vi "getY2FromFile.vi"(8 "error in (no error)":errorcluster, 10 "y2 File Name":string="y2.txt", 11 "OptCtrl in":refnum<class "OptCtrl.lvclass">) -> (0 "error out":errorcluster, 2 "y2 Matrix":dbl[][](array[numeric]), 3 "OptCtrl out":refnum<class "OptCtrl.lvclass">)   [LabVIEW 2016, in "OptCtrl.lvclass"]
doc: "Get y2 from the file. y2 is a 2D matrix (field point by z4toN)."
uses:
  OptCtrl.lvclass
  OptCtrl.lvclass/OptCtrl.ctl
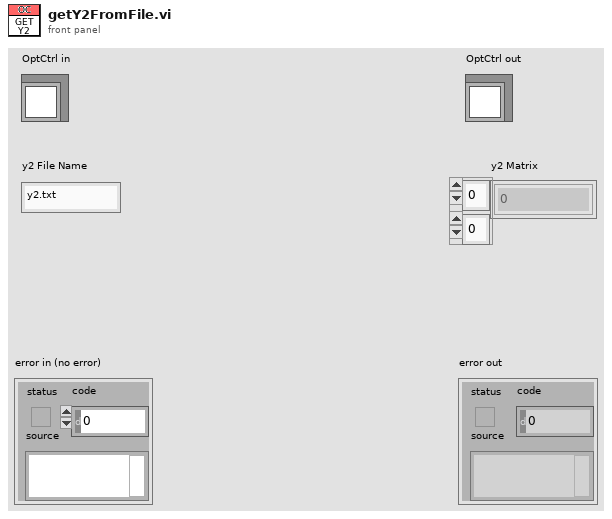
[diagram p1: front panel]
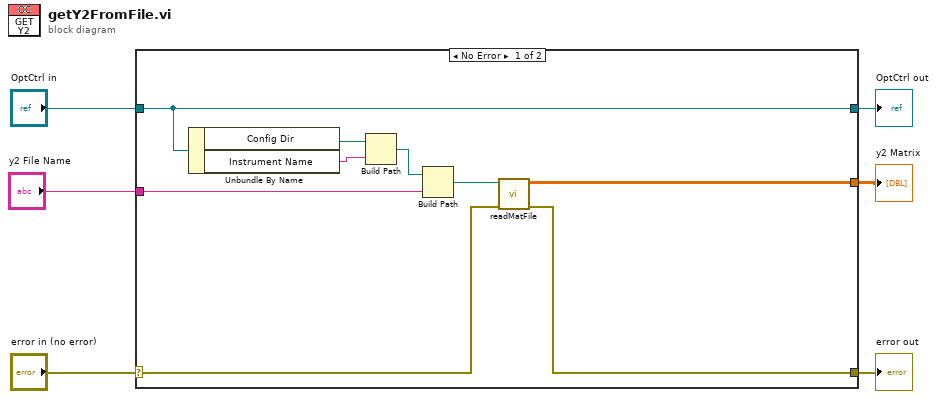
[diagram p0: block diagram]
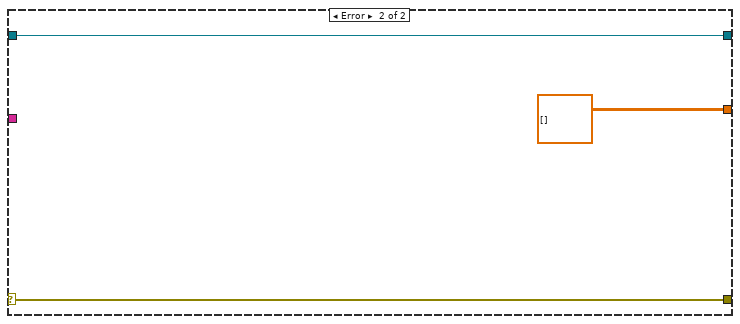
[diagram p2: hidden frame]
diagram:
  n1 = case shown="No Error" "error in (no error)" {
    selector: "error in (no error)" -> [w9 w18]
    tunnel: [w8 w18] -> w5
    tunnel: [w15 w17] -> w3
    tunnel: "OptCtrl in" -> [w15 w17]
    tunnel: "y2 File Name" -> [w11 _]
    tunnel: [w7 dbl[][] [] ("Matrix")] -> w1
    frame No Error {
      n2 = Unbundle By Name(w15) -> ("Config Dir"=w14:path, "Instrument Name"=w13:string)
      n3 = Build Path(base path=w14, name or relative path=w13) -> (appended path=w12:path)
      n4 = Build Path(base path=w12, name or relative path=w11) -> (appended path=w10:path)
      n5 = call "readMatFile.vi"("error in (no error)"=w9, "Path"=w10) -> ("error out"=w8:errorcluster, "Matrix"=w7:dbl[][])  [unwired: 8 in]
    }
    frame Error {
    }
  }
  "error out" <- w5
  "OptCtrl out" <- w3
  "y2 Matrix" <- w1
